vi "Merge Data Sets.vi"(10 "Rotation Set":T1 {"Back Right"."Angle" scale format="%.3f"; "Back Right"."Velocity" scale=-1.0..1.0 scale format="%.1f"; "Back Left"."Angle" scale format="%.3f"; "Back Left"."Velocity" scale=-1.0..1.0 scale format="%.1f"; "Front Left"."Angle" scale format="%.3f"; "Front Left"."Velocity" scale=-1.0..1.0 scale format="%.1f"; "Front Right"."Angle" scale format="%.3f"; "Front Right"."Velocity" scale=-1.0..1.0 scale format="%.1f"}, 11 "Traverse Set":T1 {"Back Right"."Angle" scale format="%.3f"; "Back Right"."Velocity" scale=-1.0..1.0 scale format="%.1f"; "Back Left"."Angle" scale format="%.3f"; "Back Left"."Velocity" scale=-1.0..1.0 scale format="%.1f"; "Front Left"."Angle" scale format="%.3f"; "Front Left"."Velocity" scale=-1.0..1.0 scale format="%.1f"; "Front Right"."Angle" scale format="%.3f"; "Front Right"."Velocity" scale=-1.0..1.0 scale format="%.1f"}) -> (2 "Calcualted Velocities Out":dbl[](array[numeric]), 3 "Swerve Data Out":T1 {"Back Right"."Angle" scale format="%.3f"; "Back Right"."Velocity" scale=-1.0..1.0 scale format="%.1f"; "Back Left"."Angle" scale format="%.3f"; "Back Left"."Velocity" scale=-1.0..1.0 scale format="%.1f"; "Front Left"."Angle" scale format="%.3f"; "Front Left"."Velocity" scale=-1.0..1.0 scale format="%.1f"; "Front Right"."Angle" scale format="%.3f"; "Front Right"."Velocity" scale=-1.0..1.0 scale format="%.1f"})   [LabVIEW 2020, in "SwerveDrive_ACT.lvlib"]
uses:
  SwerveDrive_ACT.lvlib
  Shared Code/TypeDefs/Cluster_Swerve 4 Steer and Velocity.ctl
  Shared Code/TypeDefs/Cluster_Module Velocity-Direction-Rotations.ctl
  Shared Code/TypeDefs/Level_Velocity plus-minus 1.ctl
  Shared Code/TypeDefs/Dial_Compase heading unit circle CCW positive.ctl
panel:
  # "\"Front\" of Robot"
  # "Right Hand Rule"
  # "X"
  # "+CCW"
  # "Y"
  # "(0,0)"
  # "\"Front\" of Robot"
  # "Right Hand Rule"
  # "X"
  # "+CCW"
  # "Y"
  # "(0,0)"
  # "\"Front\" of Robot"
  # "Right Hand Rule"
  # "X"
  # "+CCW"
  # "Y"
  # "(0,0)"
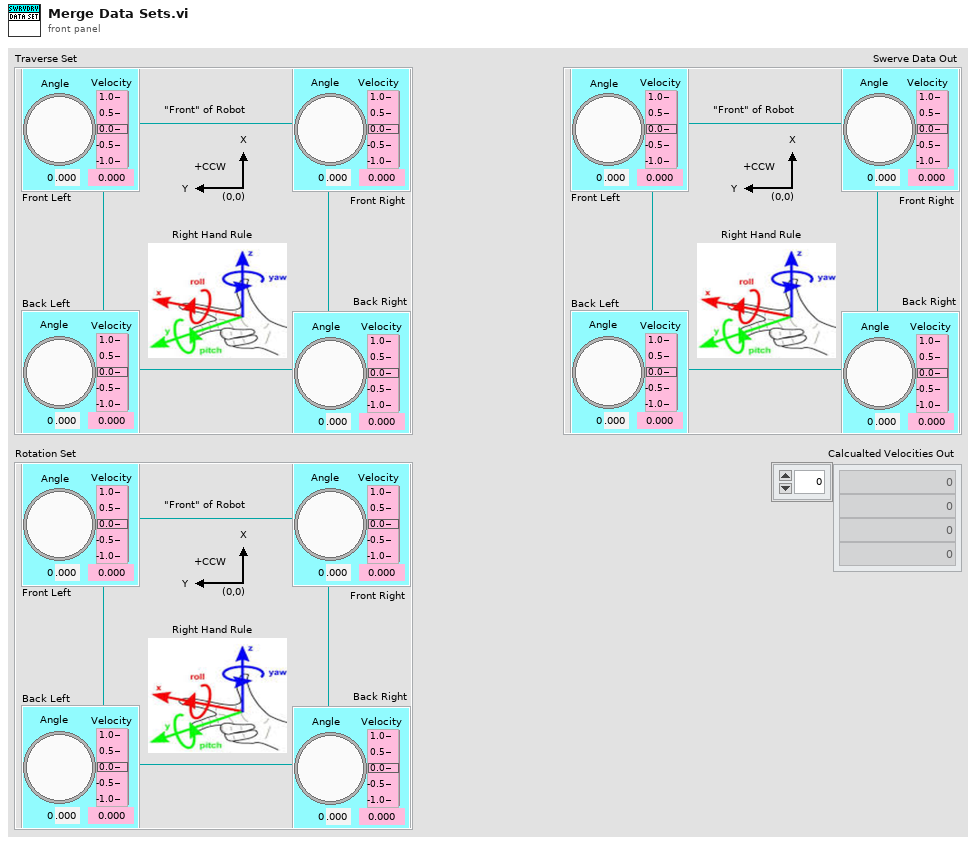
[diagram p1: front panel]
types:
  T1 = typedef "Cluster_Swerve 4 Steer and Velocity.ctl" = cluster{"Front Right":T2, "Front Left":T2, "Back Left":T2, "Back Right":T2}
  T2 = typedef "Cluster_Module Velocity-Direction-Rotations.ctl" = cluster{"Velocity":T3, "Angle":T4, "Rotations Count":dbl}
  T3 = typedef "Level_Velocity plus-minus 1.ctl" = dbl
  T4 = typedef "Dial_Compase heading unit circle CCW positive.ctl" = dbl
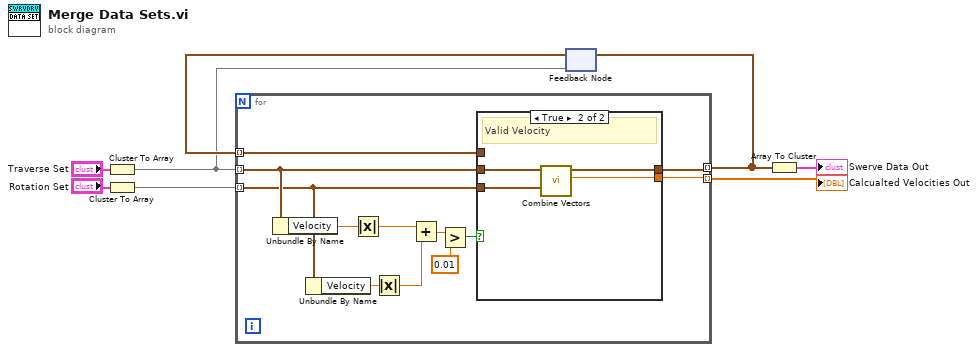
[diagram p0: block diagram]
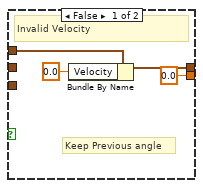
[diagram p2: hidden frame]
diagram:
  n1 = Cluster To Array(cluster="Traverse Set") -> (array=w1:T2[])
  n2 = Cluster To Array(cluster="Rotation Set") -> (array=w7:T2[])
  n3 = feedback #1(w1) -> (w2:T2[])
  n4 = for {
    tunnel: w7 -> [w18] mode=indexing
    tunnel: w1 -> [w19] mode=indexing
    tunnel: [w20] -> w5 mode=indexing
    tunnel: [w11] -> w3 mode=indexing
    tunnel: w2 -> [w12] mode=indexing
    n5 = Unbundle By Name(w19) -> ("Velocity"=w17:T3)
    n6 = Unbundle By Name(w18) -> ("Velocity"=w16:T3)
    n7 = Absolute Value(x=w17) -> (abs(x)=w10:T3)
    n8 = Absolute Value(x=w16) -> (abs(x)=w9:T3)
    n9 = Add(x=w10, y=w9) -> (x+y=w15:T3)
    n10 = Greater?(x=w15, y=T3 0.01) -> (0:w13:bool)
    n11 = case shown="True" w13 {
      tunnel: [0.0 ("Velocity Out") w28] -> w20
      tunnel: w19 -> [_ w26]
      tunnel: w18 -> [_ w25]
      tunnel: w12 -> [w21 _]
      tunnel: [w22 w27] -> w11
      frame False {
        # "Keep Previous angle"
        # "Invalid Velocity"
        n12 = Bundle By Name(cluster=w21, "Velocity"=T3 0.0) -> (w22:T2)
      }
      frame True {
        # "Valid Velocity"
        n13 = call "Combine Vectors.vi"("Rotation Module Data"=w25, "Travers Module Data"=w26) -> ("Velocity Out"=w28:dbl, "Combine Out"=w27:T2)  [unwired: 8 in]
      }
    }
  }
  "Calcualted Velocities Out" <- w5
  n14 = feedback-in #1(w3) -> ()
  n15 = Array To Cluster(array=w3) -> (cluster=→"Swerve Data Out":cluster{"[0]":T2, "[1]":T2, "[2]":T2, "[3]":T2})
